vi "testNativeXML.vi"() -> (2 "Array":string[](array[string]))   [LabVIEW 2009, in "run.lvlib"]
uses:
  Hal/testing/run.lvlib
  NativeXML.lvclass
panel:
  out "Attribute String":string
  out "Value":string
  out "Array 3":string[](array[string])
  in  "searchElementName":string
  in  "searchElementIn":string
  in  "value":string="volts"
  in  "node":string="//channel_config[@name='Ao8a_Ao_00']/mapping/units"
  out "xmlString":string
  out "Array 2":string[](array[string])
  in  "Path":path=path "C:/Documents and Settings/Administrator/Desktop/Crete/Data/Scripts/Settings Database/DeviceSettingsAtomChip.xml"
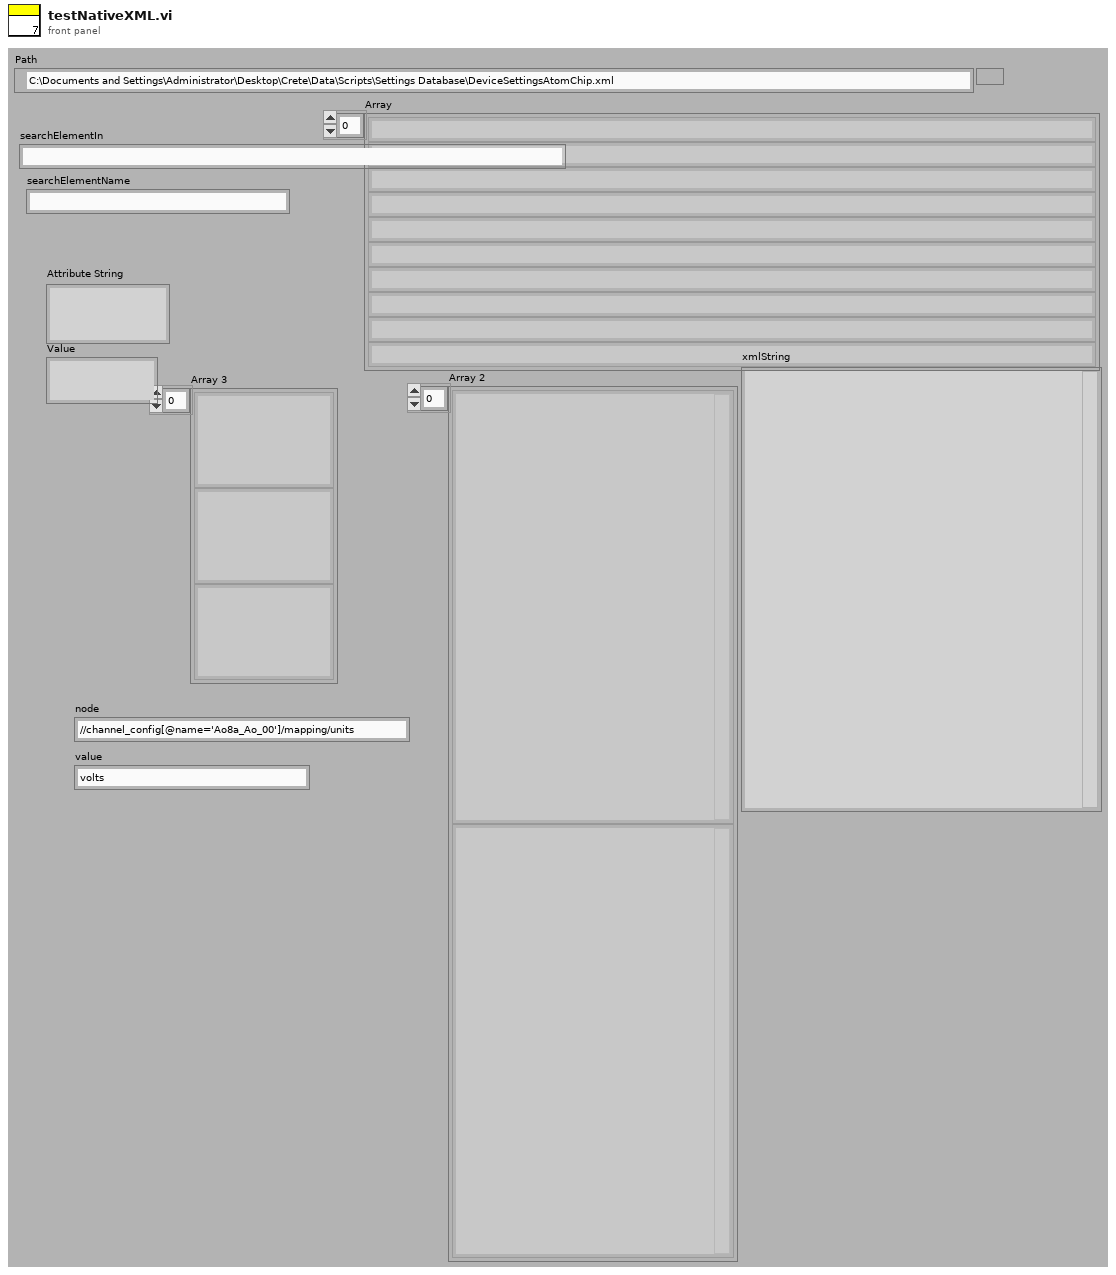
[diagram p1: front panel]
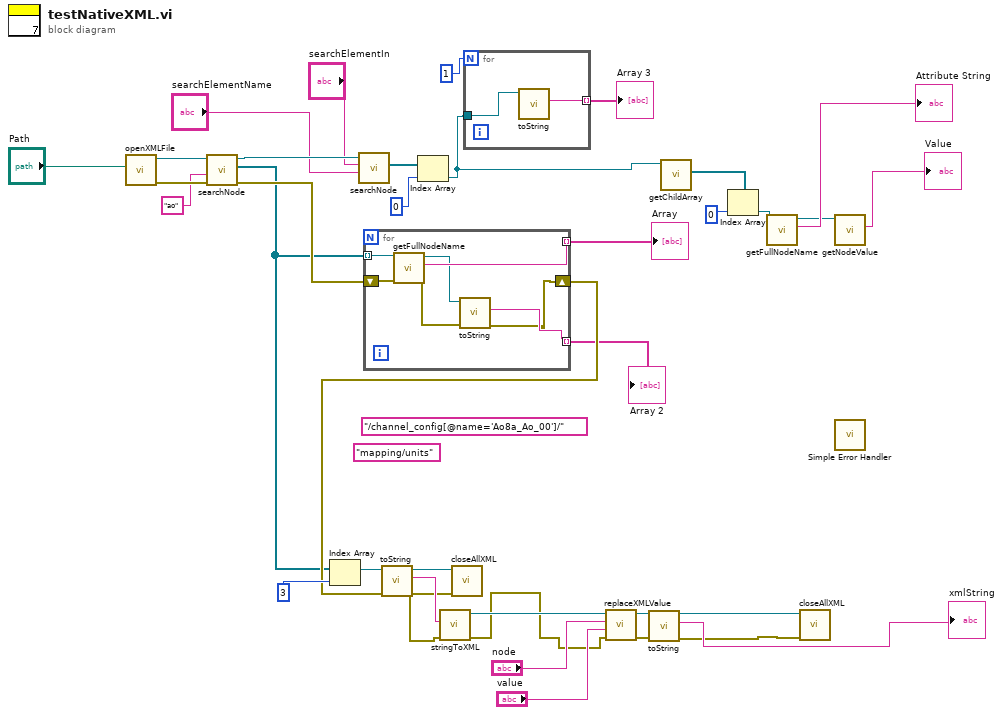
[diagram p0: block diagram]
diagram:
  (unwired) "mapping/units"
  (unwired) "/channel_config[@name='Ao8a_Ao_00']/"
  n1 = call "openXMLFile.vi"("Path"="Path") -> ("error out"=w35:errorcluster, "NativeXML out"=w36:refnum<class "NativeXML.lvclass">)  [unwired: 9 in]
  n2 = call "searchNode.vi"("error in (no error)"=w35, "searchXPath"="ao" ("searchElementName"), "NativeXML in"=w36) -> ("error out"=w20:errorcluster, "nodeArray"=w1:refnum<class "NativeXML.lvclass">[], "NativeXML out"=w16:refnum<class "NativeXML.lvclass">)  [unwired: 6 in]
  n3 = Index Array(array=w1, index=3) -> (element=w33:refnum<class "NativeXML.lvclass">)
  n4 = call "searchNode.vi"("searchXPath"="searchElementName", 10:"searchElementIn", "NativeXML in"=w16) -> ("nodeArray"=w15:refnum<class "NativeXML.lvclass">[])  [unwired: 6 in, 2 out]
  n5 = for {
    tunnel: w1 -> [w44] mode=indexing
    tunnel: [w42] -> w22 mode=indexing
    shift-right: [w38] -> w30
    shift-left: w20 -> [w43]
    tunnel: [w40] -> w21 mode=indexing
    n6 = call "getFullNodeName.vi"("error in (no error)"=w43, "NativeXML in"=w44) -> ("error out"=w39:errorcluster, "fullName"=w42:string, "NativeXML out"=w41:refnum<class "NativeXML.lvclass">)  [unwired: 7 in]
    n7 = call "toString.vi"("error in (no error)"=w39, "NativeXML in"=w41) -> ("error out"=w38:errorcluster, "xmlString"=w40:string)  [unwired: 7 in, 1 out]
  }
  "Array" <- w22
  "Array 2" <- w21
  n8 = call "toString.vi"("error in (no error)"=w30, "NativeXML in"=w33) -> ("error out"=w18:errorcluster, "xmlString"=w32:string, "NativeXML out"=w17:refnum<class "NativeXML.lvclass">)  [unwired: 7 in]
  n9 = Index Array(array=w15, index=0) -> (element=w2:refnum<class "NativeXML.lvclass">)
  n10 = call "stringToXML.vi"("error in (no error)"=w18, "xmlString"=w32) -> ("error out"=w19:errorcluster, "NativeXML out"=w28:refnum<class "NativeXML.lvclass">)  [unwired: 8 in]
  n11 = call "closeAllXML.vi"("error in (no error)"=w18, "NativeXML in"=w17) -> ()  [unwired: 9 in, 1 out]
  n12 = for {
    N: 1 -> [_]
    tunnel: w2 -> [w46]
    tunnel: [w45] -> w14 mode=indexing
    n13 = call "toString.vi"("NativeXML in"=w46) -> ("xmlString"=w45:string)  [unwired: 8 in, 2 out]
  }
  "Array 3" <- w14
  n14 = call "replaceXMLValue.vi"("error in (no error)"=w19, "value"="value", "replace in"="node", "NativeXML in"=w28) -> ("error out"=w26:errorcluster, "NativeXML out"=w25:refnum<class "NativeXML.lvclass">)  [unwired: 6 in]
  n15 = call "toString.vi"("error in (no error)"=w26, "NativeXML in"=w25) -> ("error out"=w29:errorcluster, "xmlString"=→"xmlString":string, "NativeXML out"=w23:refnum<class "NativeXML.lvclass">)  [unwired: 7 in]
  n16 = call "getChildArray.vi"("NativeXML in"=w2) -> ("childArray"=w10:refnum<class "NativeXML.lvclass">[])  [unwired: 8 in, 2 out]
  n17 = Index Array(array=w10, index=0) -> (element=w8:refnum<class "NativeXML.lvclass">)
  n18 = call "getFullNodeName.vi"("NativeXML in"=w8) -> ("fullName"=→"Attribute String":string, "NativeXML out"=w6:refnum<class "NativeXML.lvclass">)  [unwired: 8 in, 1 out]
  n19 = call "closeAllXML.vi"("error in (no error)"=w29, "NativeXML in"=w23) -> ()  [unwired: 9 in, 1 out]
  n20 = call "getNodeValue.vi"("NativeXML in"=w6) -> ("Value"=→"Value":string)  [unwired: 8 in, 2 out]
  n21 = call <vilib>:"Simple Error Handler.vi"() -> ()  [unwired: 5 in, 5 out]
